vi "4019_input_configure.vi"() -> ()   [LabVIEW 2010]
panel:
  in  "Range Setting":u16(ring)=15 items=["02     +/-100mV"=2, "03     +/-500mV"=3, "04     +/-1V"=4, "05     +/-2.5V"=5, "08     +/-10V"=8, "09     +/-5V"=9, "0D     +/-20mA"=13, "0E     Type J"=14, "0F     Type K"=15, "10     Type T"=16, "11     Type E"=17, "12     Type R"=18, "13     Type S"=19, "14     Type B"=20]
  in  "Channel":u8 max=7 step=1
  in  "Port Name":string="MainNetwork"
  in  "Use checksum":bool
  out "Reply":string
  out "?":string
  in  "Address":u8
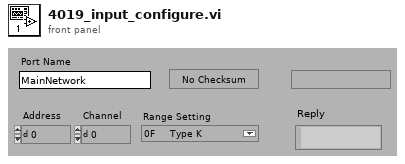
[diagram p1: front panel]
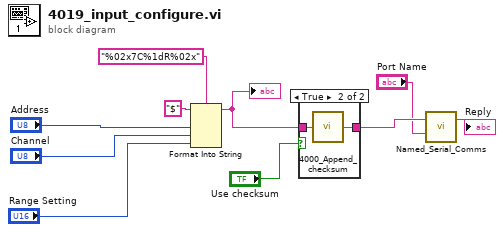
[diagram p0: block diagram]
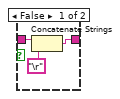
[diagram p2: hidden frame]
diagram:
  n1 = Format Into String(format string="%02x7C%1dR%02x", initial string="$", "Address", "Channel", "Range Setting") -> (resulting string=w7:string)  [unwired: 1 in, 1 out]
  "?" <- w7
  n2 = case shown="True" "Use checksum" {
    tunnel: w7 -> [w13 w15]
    tunnel: [w12 w14] -> w5
    frame False {
      n3 = Concatenate Strings(w13, "\r") -> (w12:string)
    }
    frame True {
      n4 = call "4000_Append_checksum.vi"("ADAM command"=w15) -> ("ADAM string to send"=w14:string)
    }
  }
  n5 = call "Named_Serial_Comms.vi"("Write String"=w5, "Port Name"="Port Name") -> ("Read"=→"Reply":string)  [unwired: 10 in, 3 out]
